vi "DiagnosticsCameratestglbhdl.vi"() -> ()   [LabVIEW 2010]
uses:
  Users/Public/Documents/SItoolkit/LabVIEW/Examples2010_5_0_0_0/Fast Examples/Open-Close Hardware/CamHandle.vi
panel:
  out "PvCam Minor Version":u32
  out "Major Version":u32
  out "PCI FW Ver":u32
  out "Camera FW ver":u32
  out "Camera Serial Num":u32
  out "PvCam Trivial Ver":u32
  out "Device Driver Ver":u32
  out "Internal Build":u32
  out "External Build":u32
  out "Minor Version":u32
  out "Major Version":u32
  out "Total Number of Devices":u32
  out "error out":errorcluster
  in  "error in (no error)":errorcluster
  # "Low Level Driver Version"
  # "Toolkit Version"
  # "DiagnosticsCameraTest:\n\n1.) Make sure the camera is turned on and connected."
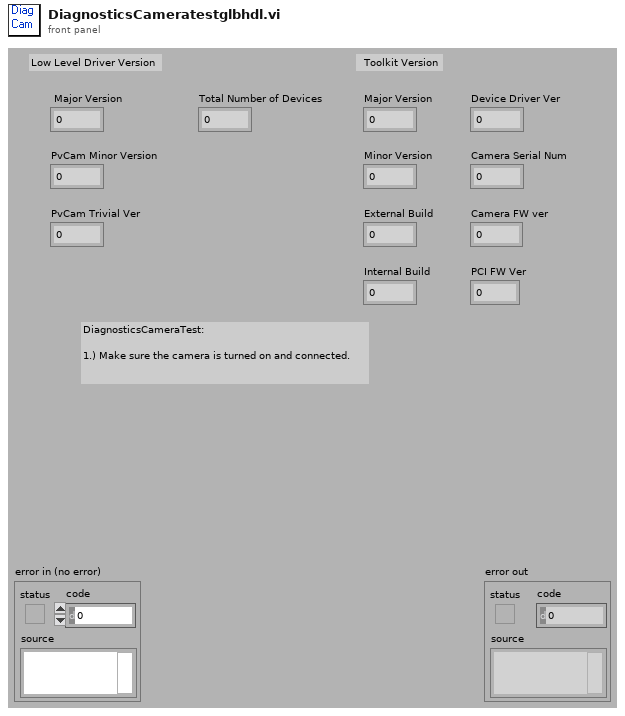
[diagram p1: front panel]
types:
  T1 = cluster{"Major Version":u32, "Minor Version":u32, "External Build":u32, "Internal Build":u32}
  T2 = cluster{"PvCam DLL Ver":u32, "Camera Serial Number ":u32, "Device Driver Ver":u32, "Camera FW Ver":u32, "PCI FW Ver":u32}
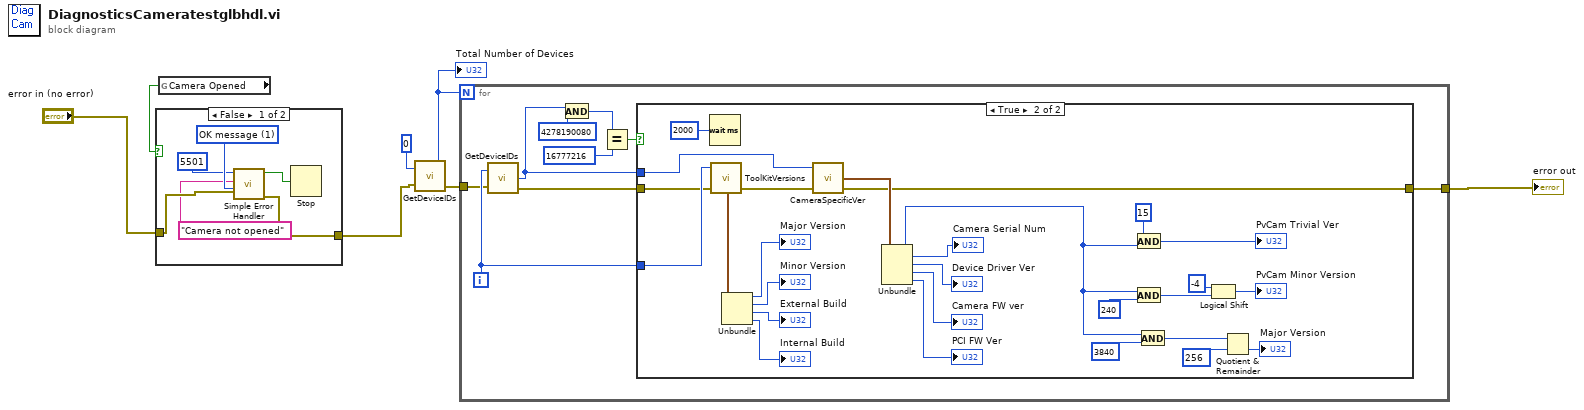
[diagram p0: block diagram]
diagram:
  n1 = global read "CamHandle.vi" "Camera Opened"() -> (w4:bool)
  n2 = case shown="False" w4 {
    tunnel: "error in (no error)" -> [w12 w14]
    tunnel: [w11 w14] -> w2
    frame False {
      w13 = u16 1 items=["no dialog", "OK message", "continue or stop message"] ("type of dialog (OK msg:1)")
      n3 = call <vilib>:"Simple Error Handler.vi"("error code (no error:0)"=5501, "error source (\" \")"="Camera not opened", "type of dialog (OK msg:1)"=w13, "error in (no error)"=w12) -> ("error?"=w9:bool, "error out"=w11:errorcluster)  [unwired: 1 in, 3 out]
      n4 = Stop(stop? (T)=w9) -> ()
    }
    frame True {
    }
  }
  n5 = call <userlib>:"GetDeviceIDs.vi"("Index"=u32 0, "error in"=w2) -> ("Total Nuber of Devices or DLLs"=w6:u32, "error out"=w5:errorcluster)  [unwired: 1 out]
  "Total Number of Devices" <- w6
  n6 = for {
    N: w6 -> [_]
    tunnel: [w21] -> w1
    tunnel: w5 -> [w19]
    i -> [w23]
    n7 = call <userlib>:"GetDeviceIDs.vi"("Index"=w23, "error in"=w19) -> ("Device ID"=w17:u32, "error out"=w18:errorcluster)  [unwired: 1 out]
    n8 = And(x=w17, y=u32 4278190080) -> (x .and. y?=w16:u32)
    n9 = Equal?(x=w16, y=u32 16777216) -> (x = y?=w20:bool)
    n10 = case shown="True" w20 {
      tunnel: w23 -> [_ w43]
      tunnel: w18 -> [w24 w27]
      tunnel: [w24 w26] -> w21
      tunnel: w17 -> [_ w25]
      frame False {
      }
      frame True {
        n11 = Wait (ms)(milliseconds to wait=u32 2000) -> ()  [unwired: 1 out]
        n12 = call <userlib>:"ToolKitVersions.vi"("error in"=w27, "Index"=w43) -> ("error out"=w42:errorcluster, "Versions"=w45:T1)  [unwired: 1 in, 1 out]
        n13 = Unbundle(w45) -> ("Major Version"=→"Major Version":u32, "Minor Version"=→"Minor Version":u32, "External Build"=→"External Build":u32, "Internal Build"=→"Internal Build":u32)
        n14 = call <userlib>:"CameraSpecificVer.vi"("error in (no error)"=w42, "Camera Handle"=w25) -> ("error out"=w26:errorcluster, "Camera Specific Versions"=w51:T2)  [unwired: 1 in, 1 out]
        n15 = Unbundle(w51) -> ("PvCam DLL Ver"=w39:u32, "Camera Serial Number"=→"Camera Serial Num":u32, "Device Driver Ver"=→"Device Driver Ver":u32, "Camera FW Ver"=→"Camera FW ver":u32, "PCI FW Ver"=→"PCI FW Ver":u32)
        n16 = And(x=u32 15, y=w39) -> (x .and. y?=→"PvCam Trivial Ver":u32)
        n17 = And(x=w39, y=u32 240) -> (x .and. y?=w29:u32)
        n18 = And(x=w39, y=u32 3840) -> (x .and. y?=w35:u32)
        n19 = Logical Shift(y=i16 -4, x=w29) -> (x << y=→"PvCam Minor Version":u32)
        n20 = Quotient & Remainder(x=w35, y=u32 256) -> (floor(x/y)=→"Major Version":u32)  [unwired: 1 out]
      }
    }
  }
  "error out" <- w1
